vi "Main.vi"(11 "Module Admin":refnum<class "Delacor_lib_QMH_Module Admin.lvclass">) -> ()   [LabVIEW 2020, in "Data Type Scripting.lvlib"]
doc: "This template is based off of the Queued Message Handler design pattern and the Queued Message Handler project template that ships with LabVIEW.\n\nThe main difference is that the queue is private to this module and communication between modules is performed via Broadcast and Request events.\n\nRequest events are wrapped in public API methods and are handled in the Event Handling Loop (EHL) of this VI. Any module can register for Broadcast events sent by this module. The EHL generates messages based on user interface actions.\n\nThe Message Handling Loop (MHL) processes messages generated by the EHL, or by other messages. The messages are string values, so new messages can be added easily to the Message Cases case structure in the MHL. Each message cluster can also provide an optional value for Message Data, which is a variant that can be converted to whatever message-specific data is required.\n_____\nBased on DQMH Project Template 6.0.0.91."
uses:
  Data Type Scripting.lvlib
  <vilib>/Delacor/Delacor QMH/Libraries/Module Admin_class/Delacor_lib_QMH_Module Admin.lvclass
  Module Data--cluster.ctl
  _td_cluster_Settings.ctl
  Support/Poly Management/_td_map_PolyRef.ctl
  Support/Poly Management/_td_map_PolyInstanceInfo.ctl
  Support/Poly Management/_td_cluster_InstanceInfo.ctl
  <vilib>/Delacor/Delacor QMH/Libraries/Message Queue_class/Delacor_lib_QMH_Message Queue.lvclass/Delacor_lib_QMH_Message Queue.ctl
  Stop Argument--cluster.ctl
  <vilib>/Delacor/Delacor QMH/Libraries/Module Admin_class/Delacor_lib_QMH_Module Admin.lvclass/Delacor_lib_QMH_Module Admin.ctl
  Load Poly VI Argument--cluster.ctl
  Get Poly List Argument--cluster.ctl
  Get Poly Details Argument--cluster.ctl
  Open Poly VI Window Argument--cluster.ctl
  Get List of Data Types Argument--cluster.ctl
  Verify New Data Type Argument--cluster.ctl
  Create New Data Type Argument--cluster.ctl
  Edit Data Type Argument--cluster.ctl
  <vilib>/Utility/miscctls.llb/LVRectTypeDef.ctl
  Remove Data Type Argument--cluster.ctl
  Open Process Data TypeDef Argument--cluster.ctl
  Close Process Data Type Def Argument--cluster.ctl
  Edit Update Data Type Argument--cluster.ctl
  <vilib>/Delacor/Delacor QMH/Libraries/Message Queue_class/Delacor_lib_QMH_Enqueue Message (Single).vi
  <vilib>/Delacor/Delacor QMH/Libraries/Module Admin_class/Delacor_lib_QMH_Get External Launch.vi
  <vilib>/Utility/error.llb/Error Cluster From Error Code.vi
  <vilib>/ErrorRing/Error Ring.xnode
  <vilib>/Delacor/Delacor QMH/Libraries/Message Queue_class/Delacor_lib_QMH_Message Queue.lvclass
panel:
  out "error out":errorcluster
  out "Status":string
  in  "Simulate MHL Error":bool
  in  "Simulate EHL Error":bool
  # "Other QMH Modules communicate with this Module via its Public API (wrappers for its Request Events).\n\nThis Module communicates with other Modules via its Broadcast Events.\nAny module that wants to get these messages, just registers for this module's Broadcast events."
  # "This template is for the Delacor Modified Queued Message Handler design pattern.\n\nSee the block diagram for more information on how to use this template."
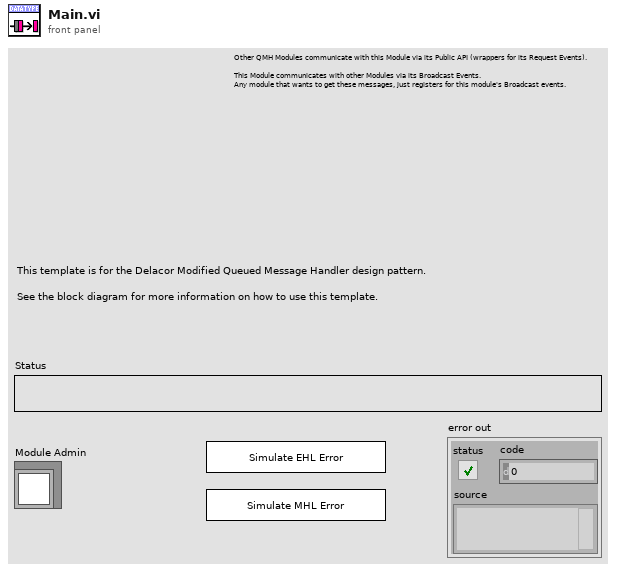
[diagram p1: front panel]
types:
  T1 = typedef "Data Type Scripting.lvlib/Request Events--cluster.ctl" = cluster{"Stop Module":refnum<user-event>, "Show Panel":refnum<user-event>, "Hide Panel":refnum<user-event>, "Get Module Execution Status":refnum<user-event>, "Show Diagram":refnum<user-event>, "Load Poly VI":refnum<user-event>, "Get Poly List":refnum<user-event>, "Get Poly Details":refnum<user-event>, "Open Poly VI Window":refnum<user-event>, "Create New Data Type":refnum<user-event>, "Verify New Data Type":refnum<user-event>, "Get List of Data Types":refnum<user-event>, "Remove Data Type":refnum<user-event>, "Open Process Data TypeDef":refnum<user-event>, "Load Edit Data Type":refnum<user-event>, "Close Process Data Type Def":refnum<user-event>, "Edit Update Data Type":refnum<user-event>}
  T2 = typedef "Data Type Scripting.lvlib/Module Data--cluster.ctl" = cluster{"Status":string, "Settings":T3, "Poly Ref Map":T4, "Poly Set Map":T5, "Valid Type?":bool, "ProcessData Ref":refnum<vi>}
  T3 = typedef "Data Type Scripting.lvlib/_td_cluster_Settings.ctl" = cluster{"NI ADAS Generic Library Path":path, "Data Types Base Directory":path, "Poly Path - Read":path, "Poly Path - Write":path, "Poly Path - Serialize":path, "Poly Path - Deserialize":path}
  T4 = typedef "_td_map_PolyRef.ctl" = map{string, refnum<vi>}
  T5 = typedef "_td_map_PolyInstanceInfo.ctl" = map{string, set{T6}}
  T6 = typedef "_td_cluster_InstanceInfo.ctl" = cluster{"VIPath":path, "Menu Name":string, "Selector Name":string}
  T7 = enum32{"invalid lock state", "Not Locked", "Locked (No Password)", "Password-protected"}
  T8 = typedef "Data Type Scripting.lvlib/Stop Argument--cluster.ctl" = cluster{"Origin":string, "Exit via Stop Module Req?":bool, "Wait for Module to stop?":bool}
  T9 = typedef "Data Type Scripting.lvlib/Load Poly VI Argument--cluster.ctl" = cluster{"Poly VI Path":path}
  T10 = typedef "Data Type Scripting.lvlib/Get Poly List Argument--cluster.ctl" = cluster{"Boolean":bool}
  T11 = typedef "Data Type Scripting.lvlib/Get Poly Details Argument--cluster.ctl" = cluster{"Poly VI Name":string}
  T12 = typedef "Data Type Scripting.lvlib/Open Poly VI Window Argument--cluster.ctl" = cluster{"Poly VI Name":string}
  T13 = typedef "Data Type Scripting.lvlib/Get List of Data Types Argument--cluster.ctl" = cluster{"Boolean":bool}
  T14 = typedef "Data Type Scripting.lvlib/Verify New Data Type Argument--cluster.ctl" = cluster{"Type Directory":path, "Type Name":string, "Menu":string, "Selector":string}
  T15 = typedef "Data Type Scripting.lvlib/Create New Data Type Argument--cluster.ctl" = cluster{"Type Directory":path, "Type Name":string, "Menu":string, "Selector":string}
  T16 = typedef "Data Type Scripting.lvlib/Edit Data Type Argument--cluster.ctl" = cluster{"Data Type":string[], "Panel Bounds":T17}
  T17 = typedef "LVRectTypeDef.ctl" = cluster{"Left":i16, "Top":i16, "Right":i16, "Bottom":i16}
  T18 = typedef "Data Type Scripting.lvlib/Remove Data Type Argument--cluster.ctl" = cluster{"Data Type to Remove":string[], "Delete Files?":bool}
  T19 = typedef "Data Type Scripting.lvlib/Open Process Data TypeDef Argument--cluster.ctl" = cluster{"Panel Bounds":T17}
  T20 = typedef "Data Type Scripting.lvlib/Close Process Data Type Def Argument--cluster.ctl" = cluster{"Boolean":bool}
  T21 = typedef "Data Type Scripting.lvlib/Edit Update Data Type Argument--cluster.ctl" = cluster{"New Data Type Name":string, "New Menu Name":string, "New Selector Name":string, "Selected Data Type":string[]}
  T22 = enum32{"Invalid", "Standard", "Closed", "Hidden", "Minimized", "Maximized"}
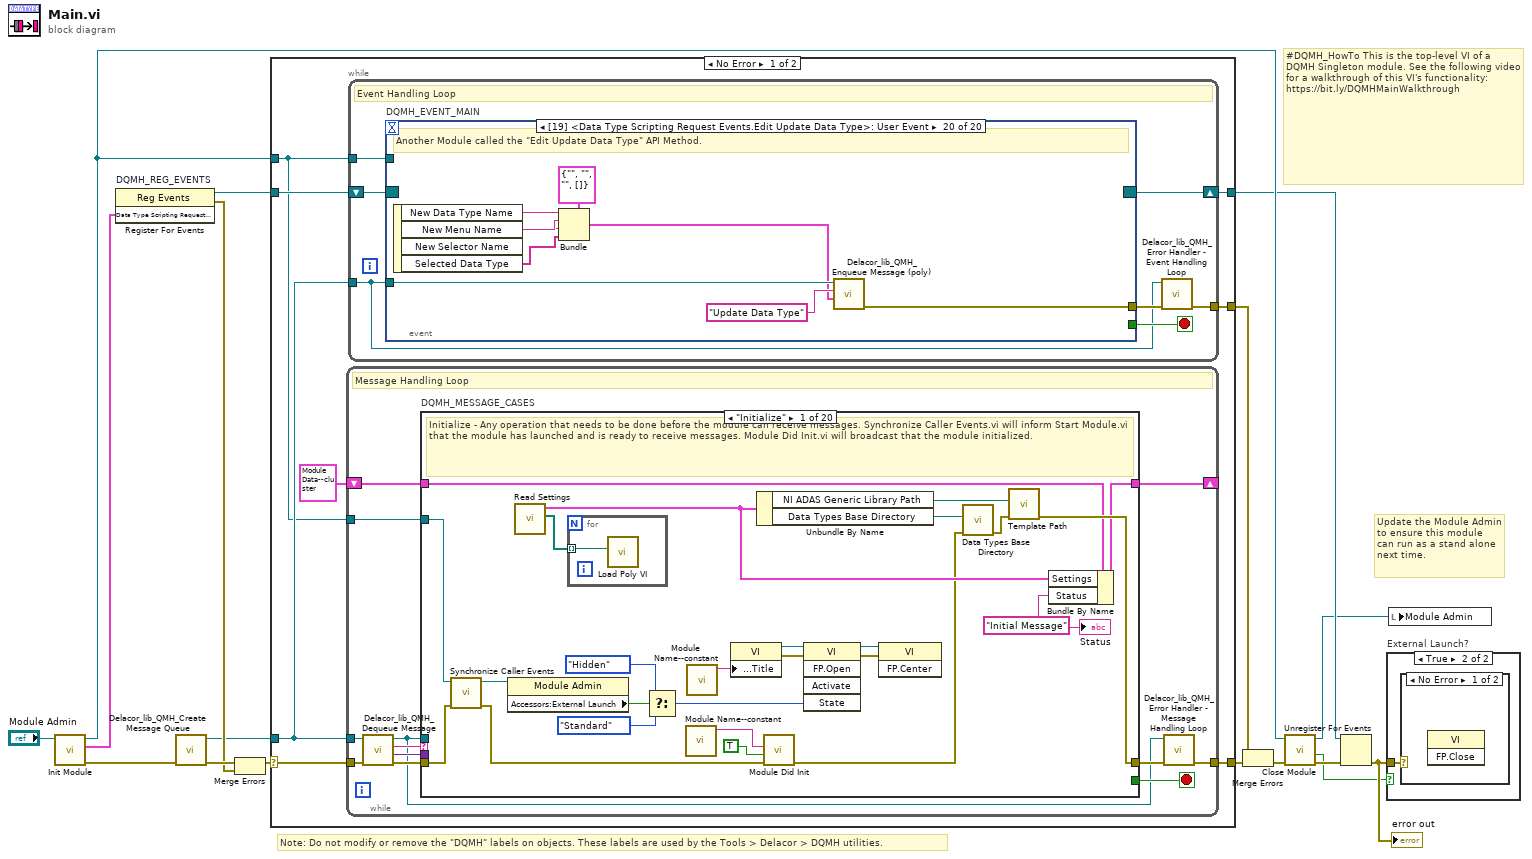
[diagram p0: block diagram]
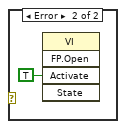
[diagram p3: hidden frame]
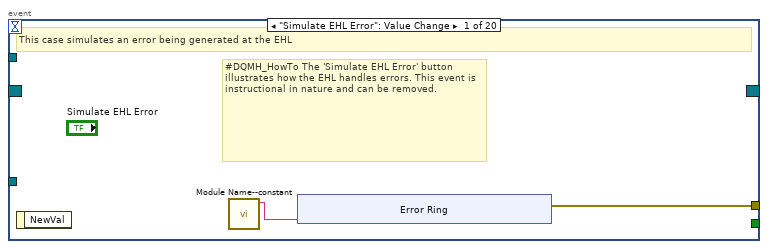
[diagram p4: hidden frame]
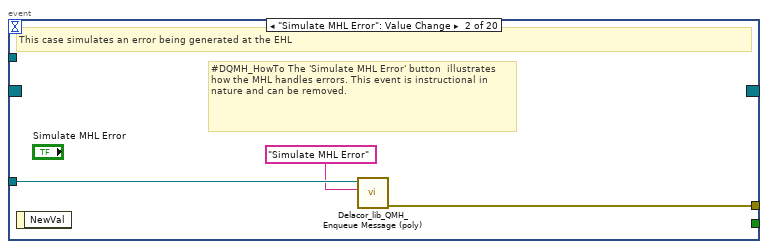
[diagram p5: hidden frame]
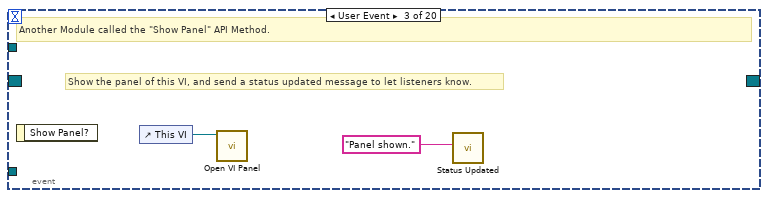
[diagram p6: hidden frame]
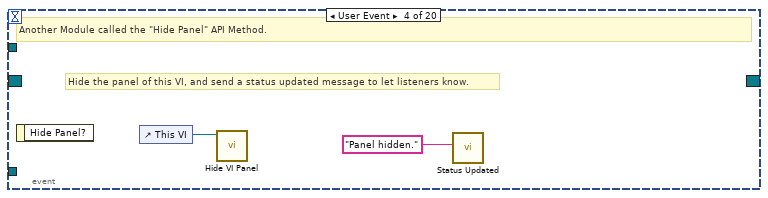
[diagram p7: hidden frame]
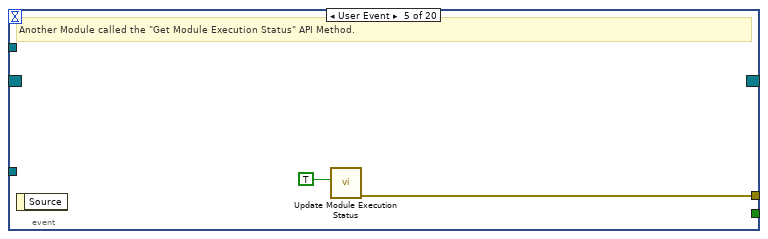
[diagram p8: hidden frame]
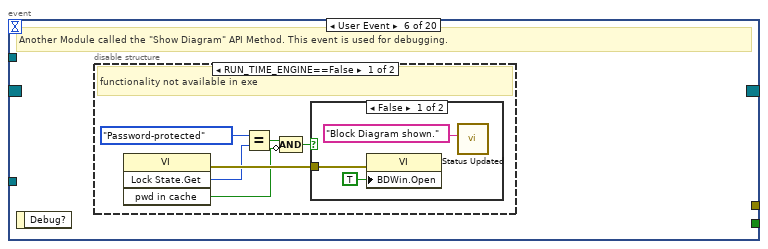
[diagram p9: hidden frame]
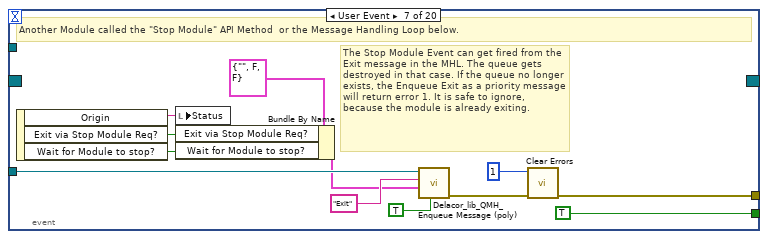
[diagram p12: hidden frame]
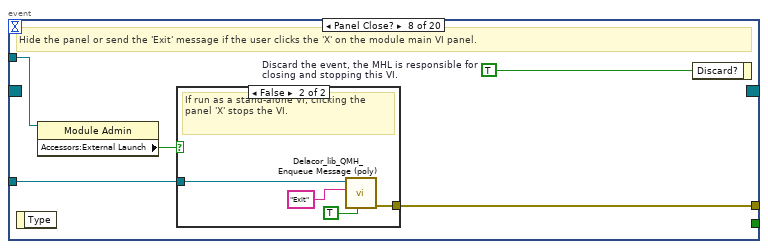
[diagram p13: hidden frame]
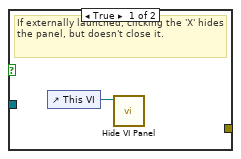
[diagram p14: hidden frame]
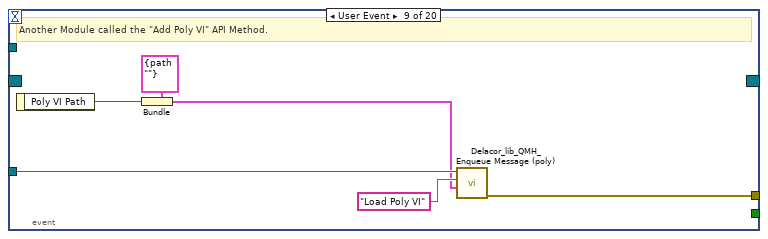
[diagram p15: hidden frame]
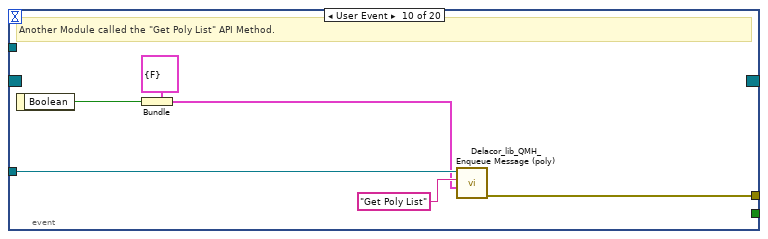
[diagram p16: hidden frame]
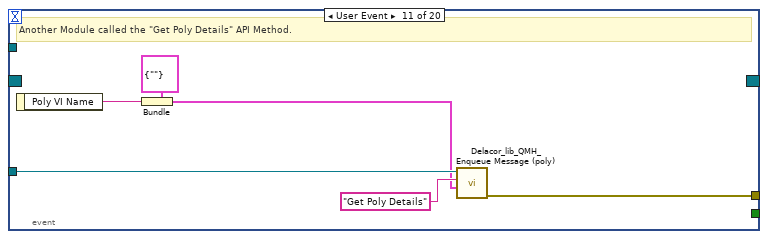
[diagram p17: hidden frame]
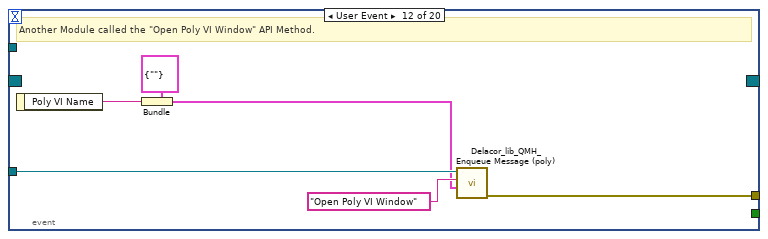
[diagram p18: hidden frame]
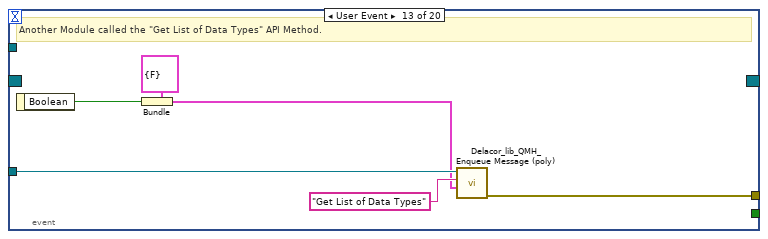
[diagram p19: hidden frame]
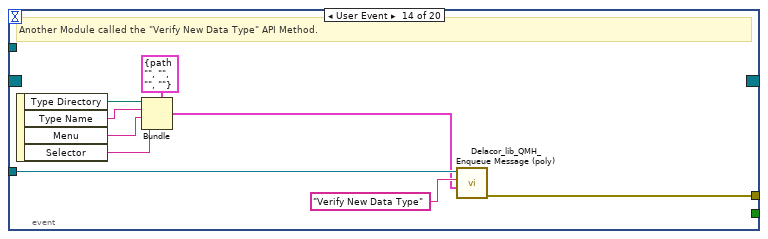
[diagram p20: hidden frame]
diagram:
  # "#DQMH_HowTo This is the top-level VI of a DQMH Singleton module. See the following video for a walkthrough of this VI's functionality: https://bit.ly/DQMHMainWalkthrough"
  # "Note: Do not modify or remove the \"DQMH\" labels on objects. These labels are used by the Tools > Delacor > DQMH utilities."
  # "Update the Module Admin to ensure this module can run as a stand alone next time."
  n1 = call "Init Module.vi"("Singleton Module Admin in"="Module Admin") -> ("error out"=w16:errorcluster, "Data Type Scripting Request Events"=w5:T1, "Singleton Module Admin out"=w8:refnum<class "Delacor_lib_QMH_Module Admin.lvclass">)  [unwired: 8 in]
  n2 = register-events "DQMH_REG_EVENTS"(w5) -> (reference out=w6:refnum<event-registration>, error out=w9:errorcluster)  [unwired: 2 in]
  n3 = call <vilib>:"Delacor_lib_QMH_Create Message Queue.vi"("error in"=w16) -> ("error out"=w11:errorcluster, "Message Queue"=w4:refnum<class "Delacor_lib_QMH_Message Queue.lvclass">)  [unwired: 9 in]
  n4 = Merge Errors(w11, w9) -> (w10:errorcluster)
  n5 = case shown="No Error" w10 {
    selector: w10 -> [w23 w477]
    tunnel: [w25 w476] -> w17
    tunnel: [w22 w482] -> w7
    tunnel: w6 -> [w20 w482]
    tunnel: w4 -> [w19 w475]
    tunnel: [w24 _] -> w14
    tunnel: w8 -> [w18 w478]
    frame No Error {
      n6 = while {
        tunnel: w19 -> [w167]
        shift-right: [w171] -> _
        shift-left: T2 {"Status"="", "Settings"={"NI ADAS Generic Library Path"=path "", "Data Types Base Directory"=path "", "Poly Path - Read"=path "", "Poly Path - Write"=path "", "Poly Path - Serialize"=path "", "Poly Path - Deserialize"=path ""}, "Poly Ref Map"={}, "Poly Set Map"={}, "Valid Type?"=FALSE, "ProcessData Ref"=refnum} ("Data Cluster") -> [w172]
        tunnel: w23 -> [w175]
        tunnel: [w173] -> w25
        tunnel: w18 -> [w165]
        stop <- w170 stop-if-true
        # "Message Handling Loop"
        n7 = call-dynamic "Delacor_lib_QMH_Dequeue Message.vi"("error in"=w175, "Message Queue in"=w167) -> ("error out"=w174:errorcluster, "Message Data"=w168:variant, "Message"=w169:string, "Message Queue out"=w166:refnum<class "Delacor_lib_QMH_Message Queue.lvclass">)  [unwired: 6 in]
        n8 = case "DQMH_MESSAGE_CASES" shown="\"Initialize\"" w169 {
          selector: w169 -> [_ _ _ _ _ _ _ _ _ _ _ _ _ _ _ _ _ _ _ w462]
          tunnel: w166 -> [_ _ _ _ _ _ _ _ _ _ _ _ _ _ _ _ _ w427 w453 _]
          tunnel: w174 -> [w198 w204 w219 w230 w246 w258 w260 w280 w292 w339 w366 w387 w392 w403 w410 w412 w417 w434 w457 w464]
          tunnel: [w201 w204 w205 w229 w237 w247 w259 w267 w291 w338 w340 w374 w394 w402 w409 w412 w416 w430 w455 w465] -> w176
          tunnel: w172 -> [w188 w203 w213 w233 w241 w254 w263 w266 w287 w321 w360 w382 w397 w401 w408 w411 w414 w429 w443 w463]
          tunnel: [w187 w203 w212 w233 w241 w254 w263 w265 w285 w326 w356 w381 w396 w400 w408 w411 w414 w429 w443 w463] -> w171
          tunnel: [_ _ _ _ _ _ _ _ _ _ _ _ _ _ _ _ _ _ w452 _] -> w170
          tunnel: w168 -> [_ _ w218 _ w245 w257 _ w279 w290 w337 w365 w386 w393 _ _ _ _ w428 w451 _]
          tunnel: w165 -> [w189 _ _ _ _ _ _ _ _ _ _ _ _ _ _ _ _ w426 w446 _]
          frame "Initialize" {
            w183 = "Initial Message" ("Initial Message")
            # "Initialize - Any operation that needs to be done before the module can receive messages. Synchronize Caller Events.vi will inform Start Module.vi that the module has launched and is ready to receive messages. Module Did Init.vi will broadcast that the module initialized."
            n9 = call "Synchronize Caller Events.vi"("error in (no error)"=w198, "Singleton Module Admin in"=w189) -> ("error out"=w197:errorcluster, "Singleton Module Admin out"=w184:refnum<class "Delacor_lib_QMH_Module Admin.lvclass">)  [unwired: 8 in]
            n10 = property class="Module Admin"(reference=w184) -> ("Accessors:External Launch"=w193:bool)  [unwired: 1 in, 2 out]
            n11 = call "Read Settings.vi"() -> ("Poly VI Paths"=w180:path[], "Settings"=w182:T3)  [unwired: 10 in]
            n12 = for {
              tunnel: w180 -> [w202] mode=indexing
              n13 = call "Load Poly VI.vi"("Poly VI Path"=w202) -> ()  [unwired: 10 in, 1 out]
            }
            n14 = Select(t=T22."Hidden" ("State"), s=w193, f=T22."Standard" ("State")) -> (s? t:f=w190:T22)
            n15 = call "Module Name--constant.vi"() -> ("Module Name"=w185:string)  [unwired: 11 in]
            n16 = call "Module Name--constant.vi"() -> ("Module Name"=w196:string)  [unwired: 11 in]
            n17 = property class="VI"("Front Panel.Title"=w196) -> (reference out=w195:refnum<vi>, error out=w200:errorcluster)  [unwired: 2 in]
            n18 = Unbundle By Name(w182) -> ("NI ADAS Generic Library Path"=w181:path, "Data Types Base Directory"=w179:path)
            n19 = call "Module Did Init.vi"("error in (no error)"=w197, "Initialized?"=TRUE, "Origin"=w185) -> ("error out"=w178:errorcluster)  [unwired: 8 in]
            n20 = invoke class="VI" method="FP.Open"(reference=w195, error in=w200, "State"=w190) -> (reference out=w194:refnum<vi>, error out=w199:errorcluster)  [unwired: 2 in, 3 out]
            n21 = invoke class="VI" method="FP.Center"(reference=w194, error in=w199) -> ()  [unwired: 1 in, 3 out]
            n22 = call "Data Types Base Directory.vi"("error in"=w178, "Data Types Directory"=w179) -> ("error out"=w177:errorcluster)  [unwired: 9 in]
            n23 = call "Template Path.vi"("error in"=w177, "Template Path"=w181) -> ("error out"=w201:errorcluster)  [unwired: 9 in]
            n24 = Bundle By Name(cluster=w188, "Settings"=w182, "Status"=w183) -> (w187:T2)
            "Status" <- w183
          }
          frame "---Module Specific---" {
            # "Separator -- The following cases handle messages specific to this Module."
          }
          frame "Load Poly VI" {
            n25 = Variant To Data(error in=w219, type=T9 {"Poly VI Path"=path ""} ("Add Poly VI Argument"), Variant=w218) -> (data=w216:T9, error out=w214:errorcluster)
            n26 = Unbundle By Name(w216) -> ("Poly VI Path"=w215:path)
            n27 = call "Open Poly VI Ref.vi"("error in"=w214, "Poly VI Path"=w215) -> ("error out"=w211:errorcluster, "Status"=w210:string, "Name"=w209:string, "Refnum out"=w208:refnum<vi>, "Success?"=w207:bool)  [unwired: 5 in]
            n28 = case shown="True" w207 {
              tunnel: w213 -> [w220 w227]
              tunnel: [w220 w226] -> w212
              tunnel: w209 -> [_ w224]
              tunnel: w208 -> [_ w221]
              frame False {
              }
              frame True {
                n29 = Unbundle By Name(w227) -> ("Poly Set Map"=w223:T5, "Poly Ref Map"=w228:T4)
                n30 = call "Poly Set Map Build.vi"("Poly Ref"=w221, "Poly Set Map in"=w223) -> ("Poly Set Map out"=w222:T5)  [unwired: 9 in]
                n31 = Insert Into Map(map in=w228, key=w224, value=w221) -> (map out=w225:T4)  [unwired: 2 out]
                n32 = Bundle By Name(cluster=w227, "Poly Set Map"=w222, "Poly Ref Map"=w225) -> (w226:T2)
              }
            }
            n33 = call "Status Updated.vi"("error in (no error)"=w211, "Status"=w210) -> ("error out"=w206:errorcluster)  [unwired: 9 in]
            n34 = call "Get Poly List.vi"("error in"=w206) -> ("error out"=w205:errorcluster)  [unwired: 10 in]
          }
          frame "Get Poly List" {
            n35 = Unbundle By Name(w233) -> ("Poly Ref Map"=w232:T4)
            n36 = for {
              tunnel: w232 -> [w236] mode=indexing
              tunnel: [w234] -> w231 mode=indexing
              n37 = Unbundle By Name(w236) -> ("Poly Ref"=w235:refnum<vi>)
              n38 = property class="PolyVI"(reference=w235) -> ("Name"=w234:string)  [unwired: 1 in, 2 out]
            }
            n39 = call "Poly List.vi"("error in"=w230, "Poly List"=w231) -> ("error out"=w229:errorcluster)  [unwired: 9 in]
          }
          frame "Get Poly Details" {
            n40 = Variant To Data(error in=w246, type=T11 {"Poly VI Name"=""} ("Get Poly Details Argument"), Variant=w245) -> (data=w243:T11, error out=w238:errorcluster)
            n41 = Unbundle By Name(w243) -> ("Poly VI Name"=w242:string)
            n42 = Unbundle By Name(w241) -> ("Poly Set Map"=w240:T5)
            n43 = call "Poly Set Map Details.vi"("Poly VI Name"=w242, "Poly Set Map in"=w240) -> ("Poly Details"=w239:T6[])  [unwired: 9 in]
            n44 = call "Poly Details.vi"("error in"=w238, "Poly Details"=w239) -> ("error out"=w237:errorcluster)  [unwired: 9 in]
          }
          frame "Open Poly VI Window" {
            n45 = Variant To Data(error in=w258, type=T12 {"Poly VI Name"=""} ("Open Poly VI Window Argument"), Variant=w257) -> (data=w255:T12, error out=w248:errorcluster)
            n46 = Unbundle By Name(w255) -> ("Poly VI Name"=w251:string)
            n47 = Unbundle By Name(w254) -> ("Poly Ref Map"=w253:T4)
            n48 = Look In Map(map=w253, key=w251) -> (value=w252:refnum<vi>)  [unwired: 1 in, 1 out]
            n49 = invoke class="PolyVI" method="FP.Open"(reference=w252) -> ()  [unwired: 4 in, 5 out]
            n50 = Format Into String(format string="Poly VI %s opened.", w251) -> (resulting string=w249:string)  [unwired: 2 in, 1 out]
            n51 = call "Status Updated.vi"("error in (no error)"=w248, "Status"=w249) -> ("error out"=w247:errorcluster)  [unwired: 9 in]
          }
          frame "Get List of Data Types" {
            n52 = Unbundle By Name(w263) -> ("Poly Set Map"=w262:T5)
            n53 = call "Poly Set Map List Data Types.vi"("Poly Set Map"=w262) -> ("Data Types"=w261:string[][])  [unwired: 10 in]
            n54 = call "List of Data Types.vi"("error in"=w260, "Data Types"=w261) -> ("error out"=w259:errorcluster)  [unwired: 9 in]
          }
          frame "Verify New Data Type" {
            n55 = Variant To Data(error in=w280, type=T14 {"Type Directory"=path "", "Type Name"="", "Menu"="", "Selector"=""} ("Verify New Data Type Argument"), Variant=w279) -> (data=w277:T14, error out=w268:errorcluster)
            n56 = Unbundle By Name(w277) -> ("Type Directory"=w276:path, "Type Name"=w275:string, "Menu"=w273:string, "Selector"=w272:string)
            n57 = Unbundle By Name(w266) -> ("Poly Set Map"=w271:T5, "Poly Ref Map"=w270:T4)
            n58 = Build Path(base path=w276, name or relative path=w275) -> (appended path=w274:path)
            n59 = call "Poly Set Map Verify New Type.vi"("Poly Set Map"=w271, "Poly Ref Map"=w270, "Selector Name"=w272, "Menu Name"=w273, "Directory"=w274) -> ("Valid?"=w264:bool, "Error Message"=w269:string)  [unwired: 5 in]
            n60 = call "Data Type Valid.vi"("error in"=w268, "Valid"=w264, "Error Msg"=w269) -> ("error out"=w267:errorcluster)  [unwired: 8 in]
            n61 = Bundle By Name(cluster=w266, "Valid Type?"=w264) -> (w265:T2)
          }
          frame "Create New Data Type" {
            n62 = Unbundle By Name(w287) -> ("Poly Ref Map"=w288:T4, "Poly Set Map"=w289:T5, "Settings.NI ADAS Generic Library Path"=w283:path, "Valid Type?"=w284:bool, "ProcessData Ref"=w282:refnum<vi>)
            n63 = case shown="True" w284 {
              tunnel: w292 -> [w295 w315]
              tunnel: [w295 w297] -> w291
              tunnel: w290 -> [_ w314]
              tunnel: w289 -> [w294 w311]
              tunnel: w288 -> [_ w310]
              tunnel: [w294 w307] -> w286
              tunnel: w283 -> [_ w306]
              tunnel: w282 -> [w293 w302]
              tunnel: [w293 refnum<vi> refnum ("ProcessData Ref")] -> w281
              frame False {
              }
              frame True {
                n64 = Variant To Data(error in=w315, type=T15 {"Type Directory"=path "", "Type Name"="", "Menu"="", "Selector"=""} ("Create New Data Type Argument"), Variant=w314) -> (data=w312:T15)  [unwired: 1 out]
                n65 = Unbundle By Name(w312) -> ("Type Directory"=w299:path, "Type Name"=w305:string, "Menu"=w308:string, "Selector"=w309:string)
                n66 = call "Copy Library.vi"("New Name"=w305, "Destination Directory"=w299, "Path to Library"=w306) -> ("error out"=w304:errorcluster, "New Library Path"=w296:path)  [unwired: 7 in]
                n67 = call "Poly Set Map Add New Type.vi"("Selector Name"=w309, "Poly Ref Map"=w310, "error in (no error)"=w304, "Menu Name"=w308, "New Library Path"=w296, "Poly Map Set in"=w311) -> ("error out"=w303:errorcluster, "Poly Map Set out"=w307:T5)  [unwired: 4 in]
                n68 = call "Save Process Data TypeDef.vi"("error in (no error)"=w303, "Path to Library"=w296, "ProcessData Ref"=w302) -> ("error out"=w300:errorcluster)  [unwired: 8 in]
                n69 = call "Update test_serialize_deserialize.vi"("error in (no error)"=w300, "Path to Library"=w296) -> ("error out"=w298:errorcluster)  [unwired: 9 in]
                n70 = call "Data Type Created.vi"("error in"=w298, "Path"=w296) -> ("error out"=w297:errorcluster)  [unwired: 9 in]
              }
            }
            n71 = Bundle By Name(cluster=w287, "Poly Set Map"=w286, "ProcessData Ref"=w281) -> (w285:T2)
          }
          frame "Load Edit Data Type" {
            n72 = Unbundle By Name(w321) -> ("ProcessData Ref"=w318:refnum<vi>)
            n73 = Variant To Data(error in=w339, type=T16 {"Data Type"=[], "Panel Bounds"={"Left"=0, "Top"=0, "Right"=0, "Bottom"=0}} ("Edit Data Type Argument"), Variant=w337) -> (data=w335:T16, error out=w338:errorcluster)
            n74 = Unbundle By Name(w335) -> ("Panel Bounds"=w316:T17, "Data Type"=w330:string[])
            n75 = invoke class="VI" method="FP.Close"(reference=w318) -> (reference out=w317:refnum<vi>)  [unwired: 2 in, 2 out]
            n76 = Close Reference(reference=w317) -> (error out=w320:errorcluster)  [unwired: 1 in]
            n77 = call <vilib>:"Clear Errors.vi"("error in (no error)"=w320) -> ("error out"=w319:errorcluster)  [unwired: 5 in, 1 out]
            n78 = Index Array(array=w330, index #1=0 ("index"), index #2=1 ("index"), index #3=2 ("index")) -> (element #1=w325:string, element #2=w324:string, element #3=w332:string)
            n79 = String To Path(string=w332) -> (path=w323:path)
            n80 = Build Path(base path=w323, name or relative path="Process Data.ctl") -> (appended path=w327:path)
            n81 = Strip Path(path=w323) -> (name=w322:string)  [unwired: 1 out]
            n82 = call "Open Process Data TypeDef.vi"("error in (no error)"=w319, "Panel Bounds"=w316, "Path to Library"=w327) -> ("ProcessData Ref"=w328:refnum<vi>)  [unwired: 7 in, 1 out]
            n83 = call "Selected Edit Data Type Info.vi"("Selector Name"=w325, "Menu Name"=w324, "Data Type Name"=w322) -> ()  [unwired: 8 in, 1 out]
            n84 = Bundle By Name(cluster=w321, "ProcessData Ref"=w328) -> (w326:T2)
          }
          frame "Update Data Type" {
            # "Don't delete if user\ndidn't change name"
            n85 = Variant To Data(error in=w366, type=T21 {"New Data Type Name"="", "New Menu Name"="", "New Selector Name"="", "Selected Data Type"=[]} ("Edit Update Data Type Argument"), Variant=w365) -> (data=w363:T21, error out=w352:errorcluster)
            n86 = Unbundle By Name(w363) -> ("Selected Data Type"=w362:string[], "New Data Type Name"=w346:string, "New Menu Name"=w355:string, "New Selector Name"=w354:string)
            n87 = Unbundle By Name(w360) -> ("Poly Ref Map"=w358:T4, "ProcessData Ref"=w353:refnum<vi>, "Poly Set Map"=w343:T5)
            n88 = call "Poly Set Map Remove Type.vi"("Poly Ref Map"=w358, "error in (no error)"=w352, "Delete Files?"=FALSE, "Data Type to Remove"=w362, "Poly Set Map in"=w343) -> ("error out"=w351:errorcluster, "Data Type Library Path"=w349:path, "Data Type Directory"=w347:path, "Poly Set Map out"=w359:T5)  [unwired: 3 in]
            n89 = call "Save Process Data TypeDef.vi"("error in (no error)"=w351, "Path to Library"=w349, "ProcessData Ref"=w353) -> ("error out"=w350:errorcluster)  [unwired: 8 in]
            n90 = Strip Path(path=w347) -> (name=w345:string)  [unwired: 1 out]
            n91 = Not Equal?(x=w346, y=w345) -> (x != y?=w344:bool)
            n92 = call "Edit - Data Type Library.vi"("Data Type Directory"=w347, "Data Type Library Path"=w349, "New Data Type Name"=w346, "error in"=w350) -> ("New Data Type Library Path"=w342:path, "Old Directory to Delete"=w348:path, "error out"=w367:errorcluster)  [unwired: 9 in]
            n93 = call "Poly Set Map Add New Type.vi"("Selector Name"=w354, "Poly Ref Map"=w358, "error in (no error)"=w367, "Menu Name"=w355, "New Library Path"=w342, "Poly Map Set in"=w359) -> ("error out"=w368:errorcluster, "Poly Map Set out"=w357:T5)  [unwired: 4 in]
            n94 = case shown="True" w344 {
              tunnel: w348 -> [_ w373]
              tunnel: w368 -> [w369 w372]
              tunnel: [w369 w371] -> w341
              frame False {
              }
              frame True {
                n95 = Delete(path (use dialog)=w373, entire hierarchy (F)=TRUE, error in=w372) -> (error out=w371:errorcluster)  [unwired: 2 in, 2 out]
              }
            }
            n96 = Bundle By Name(cluster=w360, "Poly Set Map"=w357) -> (w356:T2)
            n97 = call "Data Type Updated.vi"("error in"=w341, "Data Type Library Path"=w342) -> ("error out"=w340:errorcluster)  [unwired: 9 in]
          }
          frame "Remove Data Type" {
            n98 = Variant To Data(error in=w387, type=T18 {"Data Type to Remove"=[], "Delete Files?"=FALSE} ("Remove Data Type Argument"), Variant=w386) -> (data=w384:T18, error out=w375:errorcluster)
            n99 = Unbundle By Name(w382) -> ("Poly Ref Map"=w383:T4, "Poly Set Map"=w380:T5)
            n100 = Unbundle By Name(w384) -> ("Data Type to Remove"=w378:string[], "Delete Files?"=w377:bool)
            n101 = call "Poly Set Map Remove Type.vi"("Poly Ref Map"=w383, "error in (no error)"=w375, "Delete Files?"=w377, "Data Type to Remove"=w378, "Poly Set Map in"=w380) -> ("error out"=w376:errorcluster, "Poly Set Map out"=w379:T5)  [unwired: 3 in, 2 out]
            n102 = Bundle By Name(cluster=w382, "Poly Set Map"=w379) -> (w381:T2)
            n103 = call "Get List of Data Types.vi"("error in"=w376) -> ("error out"=w374:errorcluster)  [unwired: 10 in]
          }
          frame "Open Process Data TypeDef" {
            n104 = Variant To Data(error in=w392, type=T19 {"Panel Bounds"={"Left"=0, "Top"=0, "Right"=0, "Bottom"=0}} ("Open Process Data TypeDef Argument"), Variant=w393) -> (data=w390:T19, error out=w388:errorcluster)
            n105 = Unbundle By Name(w397) -> ("Settings.NI ADAS Generic Library Path"=w398:path)
            n106 = Unbundle By Name(w390) -> ("Panel Bounds"=w389:T17)
            n107 = call "Open Process Data TypeDef.vi"("error in (no error)"=w388, "Panel Bounds"=w389, "Path to Library"=w398) -> ("error out"=w394:errorcluster, "ProcessData Ref"=w395:refnum<vi>)  [unwired: 7 in]
            n108 = Bundle By Name(cluster=w397, "ProcessData Ref"=w395) -> (w396:T2)
          }
          frame "Close Process Data Type Def" {
            n109 = Unbundle By Name(w401) -> ("ProcessData Ref"=w404:refnum<vi>)
            n110 = invoke class="VI" method="FP.Close"(reference=w404, error in=w403) -> (reference out=w406:refnum<vi>, error out=w405:errorcluster)  [unwired: 1 in, 1 out]
            n111 = Close Reference(reference=w406, error in (no error)=w405) -> (error out=w407:errorcluster)
            n112 = call <vilib>:"Clear Errors.vi"("error in (no error)"=w407) -> ("error out"=w402:errorcluster)  [unwired: 5 in, 1 out]
            n113 = Bundle By Name(cluster=w401, "ProcessData Ref"=refnum<vi> refnum) -> (w400:T2)
          }
          frame "---Copy This Frame---" {
            # "Duplicate this frame when creating new messages.  Change this comment in the duplicated frame to describe this message."
            n114 = Merge Errors(w410) -> (w409:errorcluster)
          }
          frame "---Exit and Error Handling---" {
            # "Separator - The following cases handle errors and exit messages."
          }
          frame "Simulate MHL Error" {
            # "#DQMH_HowTo The 'Simulate MHL Error' button  illustrates how the MHL handles errors. This event is instructional in nature and can be removed."
            # "Simulate an error occurring at the MHL"
            n115 = call "Module Name--constant.vi"() -> ("Module Name"=w413:string)  [unwired: 11 in]
            n116 = xnode "Error Ring"("parameter 0"=w413) -> ("error out"=w415:errorcluster)
            n117 = Merge Errors(w417, w415) -> (w416:errorcluster)
          }
          frame "Error" {
            # "#CodeRecommended - If you ever change the name of this \"Error\" message, you'll need to update the name in the Check Loop Error.vi as well."
            # "#CodeRecommended - If the module is running in standalone mode (External Launch = FALSE), this code will pop up an error dialog and call the 'Exit' message if an error occurs. Add more fine-grained error handling here."
            # "Error - Check the error message data and respond accordingly. This message is sent by the \"Error Handler\" VIs at the end of each loop in this application."
            n118 = property class="Module Admin"(reference=w426) -> ("Accessors:External Launch"=w425:bool)  [unwired: 1 in, 2 out]
            n119 = Variant To Data(error in=w434, type=errorcluster {"status"=FALSE, "code"=0, "source"=""} ("error constant"), Variant=w428) -> (data=w435:errorcluster, error out=w432:errorcluster)
            n120 = call "Error Reported.vi"("Error"=w435) -> ()  [unwired: 10 in, 1 out]
            n121 = case shown="False" w425 {
              tunnel: [w440 _] -> w431
              tunnel: w427 -> [w438 _]
              tunnel: w435 -> [w439 _]
              frame False {
                # "If the module is running standalone, then pop up an error dialog and call the \"Exit\" message."
                n122 = call <vilib>:"Simple Error Handler.vi"("error in (no error)"=w439) -> ()  [unwired: 4 in, 5 out]
                n123 = call-poly <vilib>:"Delacor_lib_QMH_Enqueue Message (poly).vi"("Priority Message? (F)"=TRUE, "Message"="Exit", "Message Queue in"=w438) -> ("error out"=w440:errorcluster)  [unwired: 7 in, 1 out]
              }
              frame True {
                # "If the module was launched externally, calling the Error Reported broadcast VI is the only action performed by the \"Error\" message. The module's caller can then process the error appropriately."
              }
            }
            n124 = Merge Errors(w432, w431) -> (w430:errorcluster)
            n125 = local write "error out"(w430) -> ()
          }
          frame "Exit" {
            w450 = 91  # 91: not all Exit messages will have an argument
            w452 = TRUE  # Stop the VI
            # "Release the message queue reference"
            # "Exit - Exit the application."
            n126 = control-ref of="This VI"() -> (w447:refnum<vi>)
            n127 = Variant To Data(error in=w457, type=T8 {"Origin"="", "Exit via Stop Module Req?"=FALSE, "Wait for Module to stop?"=FALSE} ("Stop Argument"), Variant=w451) -> (data=w448:T8, error out=w454:errorcluster)
            n128 = call "Handle Exit.vi"("Stop Argument"=w448, "Admin in"=w446, "VI reference"=w447) -> ("error out"=w445:errorcluster)  [unwired: 7 in, 1 out]
            n129 = call <vilib>:"Clear Errors.vi"("error in (no error)"=w454, "specific error code to clear (0: all)"=w450) -> ("error out"=w456:errorcluster)  [unwired: 4 in, 1 out]
            n130 = call-dynamic "Delacor_lib_QMH_Release Message Queue.vi"("error in"=w456, "Message Queue"=w453) -> ("error out"=w444:errorcluster)  [unwired: 9 in]
            n131 = Unbundle By Name(w443) -> ("Poly Ref Map"=w442:T4)
            n132 = for {
              tunnel: w442 -> [w460] mode=indexing
              tunnel: [w458] -> w441 mode=indexing
              n133 = Unbundle By Name(w460) -> ("Poly Ref"=w459:refnum<vi>)
              n134 = Close Reference(reference=w459) -> (error out=w458:errorcluster)  [unwired: 1 in]
            }
            n135 = Merge Errors(w441, w445, w444) -> (w455:errorcluster)
          }
          frame Default {
            # "'Default' case only runs if there is a message that isn't defined in any of the other cases.  Output a programming error."
            n136 = call "Module Name--constant.vi"() -> ("Module Name"=w461:string)  [unwired: 11 in]
            n137 = xnode "Error Ring"("parameter 0"=w462, "parameter 1"=w461) -> ("error out"=w466:errorcluster)
            n138 = Merge Errors(w464, w466) -> (w465:errorcluster)
          }
        }
        n139 = call-dynamic "Delacor_lib_QMH_Error Handler - Message Handling Loop.vi"("error in"=w176, "Message Queue in"=w166) -> ("dup error in"=w173:errorcluster)  [unwired: 8 in, 1 out]
      }
      n140 = while {
        tunnel: w19 -> [w26]
        shift-right: [w29] -> w22
        shift-left: w20 -> [w30]
        tunnel: [w31] -> w24
        tunnel: w18 -> [w27]
        stop <- w28 stop-if-true
        # "Event Handling Loop"
        n141 = event "DQMH_EVENT_MAIN" shown="[19] <Data Type Scripting Request Events.Edit Update Data Type>: User Event" {
          selector: w30 -> [_ _ _ _ _ _ _ _ _ _ _ _ _ _ _ _ _ _ _ _]
          dyn-events: [_ _ _ _ _ _ _ _ _ _ _ _ _ _ _ _ _ _ _ _] -> w29
          timeout: _ -> [_ _ _ _ _ _ _ _ _ _ _ _ _ _ _ _ _ _ _ _]
          tunnel: [_ _ _ _ _ _ TRUE ("Discard?") _ _ _ _ _ _ _ _ _ _ _ _ _] -> w28
          tunnel: w26 -> [_ w43 _ _ _ _ w67 w74 w87 w93 w99 w105 w111 w120 w129 w136 w143 w149 w155 w164]
          tunnel: [w34 w44 _ _ w50 _ w70 w76 w82 w88 w94 w100 w106 w112 w121 w131 w137 w145 w150 w156] -> w32
          tunnel: w27 -> [_ _ _ _ _ _ _ w73 _ _ _ _ _ _ _ _ _ _ _ _]
          event "Simulate EHL Error": Value Change {
            # "#DQMH_HowTo The 'Simulate EHL Error' button  illustrates how the EHL handles errors. This event is instructional in nature and can be removed."
            # "This case simulates an error being generated at the EHL"
            n142 = event-data() -> ()  [unwired: 1 in, 1 out]
            n143 = call "Module Name--constant.vi"() -> ("Module Name"=w33:string)  [unwired: 11 in]
            n144 = xnode "Error Ring"("parameter 0"=w33) -> ("error out"=w34:errorcluster)
          }
          event "Simulate MHL Error": Value Change {
            # "#DQMH_HowTo The 'Simulate MHL Error' button  illustrates how the MHL handles errors. This event is instructional in nature and can be removed."
            # "This case simulates an error being generated at the EHL"
            n145 = event-data() -> ()  [unwired: 1 in, 1 out]
            n146 = call-poly <vilib>:"Delacor_lib_QMH_Enqueue Message (poly).vi"("Message"="Simulate MHL Error", "Message Queue in"=w43) -> ("error out"=w44:errorcluster)  [unwired: 8 in, 1 out]
          }
          event User Event {
            # "Show the panel of this VI, and send a status updated message to let listeners know."
            # "Another Module called the \"Show Panel\" API Method."
            n147 = event-data() -> ()  [unwired: 1 in, 1 out]
            n148 = control-ref of="This VI"() -> (w46:refnum<vi>)
            n149 = call "Open VI Panel.vi"("VI"=w46) -> ()  [unwired: 10 in, 1 out]
            n150 = call "Status Updated.vi"("Status"="Panel shown." ("format string")) -> ()  [unwired: 10 in, 1 out]
          }
          event User Event {
            # "Hide the panel of this VI, and send a status updated message to let listeners know."
            # "Another Module called the \"Hide Panel\" API Method."
            n151 = event-data() -> ()  [unwired: 1 in, 1 out]
            n152 = control-ref of="This VI"() -> (w48:refnum<vi>)
            n153 = call "Hide VI Panel.vi"("VI"=w48) -> ()  [unwired: 10 in, 1 out]
            n154 = call "Status Updated.vi"("Status"="Panel hidden." ("format string")) -> ()  [unwired: 10 in, 1 out]
          }
          event User Event {
            # "Another Module called the \"Get Module Execution Status\" API Method."
            n155 = event-data() -> ()  [unwired: 1 in, 1 out]
            n156 = call "Update Module Execution Status.vi"("Running?"=TRUE) -> ("error out"=w50:errorcluster)  [unwired: 10 in]
          }
          event User Event {
            # "Another Module called the \"Show Diagram\" API Method. This event is used for debugging."
            n157 = event-data() -> ()  [unwired: 1 in, 1 out]
            n158 = disable-structure shown="RUN_TIME_ENGINE==False" {
              frame condition #0 (active) {
                # "functionality not available in exe"
                n159 = invoke class="VI" method="Lock State.Get"() -> (error out=w56:errorcluster, "Get Lock State"=w55:T7, "pwd in cache"=w52:bool)  [unwired: 4 in, 1 out]
                n160 = Equal?(x=T7."Password-protected", y=w55) -> (x = y?=w53:bool)
                n161 = Compound Arithmetic op=AND(w53, invert w52) -> (w51:bool)
                n162 = case shown="False" w51 {
                  tunnel: w56 -> [w59 _]
                  frame False {
                    n163 = property class="VI"(error in=w59, "BDWin.Open"=TRUE ("Block Diagram Window:Open")) -> ()  [unwired: 1 in, 2 out]
                    n164 = call "Status Updated.vi"("Status"="Block Diagram shown." ("format string")) -> ()  [unwired: 10 in, 1 out]
                  }
                  frame True {
                    # "Password-protected VI, and the password is not in the cache. Do not show the diagram."
                  }
                }
              }
              frame condition #1 {
              }
            }
          }
          event User Event {
            # "The Stop Module Event can get fired from the Exit message in the MHL. The queue gets destroyed in that case. If the queue no longer exists, the Enqueue Exit as a priority message will return error 1. It is safe to ignore, because the module is already exiting."
            # "Another Module called the \"Stop Module\" API Method  or the Message Handling Loop below."
            n165 = event-data() -> ("Origin"=w66:string, "Exit via Stop Module Req?"=w62:bool, "Wait for Module to stop?"=w61:bool)  [unwired: 1 in]
            n166 = local write "Status"(w66) -> ()
            n167 = Bundle By Name(cluster=T8 {"Origin"="", "Exit via Stop Module Req?"=FALSE, "Wait for Module to stop?"=FALSE} ("Stop Argument"), "Exit via Stop Module Req?"=w62, "Wait for Module to stop?"=w61) -> (w60:T8)
            n168 = call-poly <vilib>:"Delacor_lib_QMH_Enqueue Message (poly).vi"("Priority Message? (F)"=TRUE, "Message Data"=w60, "Message"="Exit", "Message Queue in"=w67) -> ("error out"=w71:errorcluster)  [unwired: 6 in, 1 out]
            n169 = call <vilib>:"Clear Errors.vi"("error in (no error)"=w71, "specific error code to clear (0: all)"=1) -> ("error out"=w70:errorcluster)  [unwired: 4 in, 1 out]
          }
          event Panel Close? {
            w75 = TRUE  # Discard the event, the MHL is responsible for closing and stopping this VI.
            # "Hide the panel or send the 'Exit' message if the user clicks the 'X' on the module main VI panel."
            n170 = event-data() -> ()  [unwired: 1 in, 1 out]
            n171 = property class="Module Admin"(reference=w73) -> ("Accessors:External Launch"=w72:bool)  [unwired: 1 in, 2 out]
            n172 = case shown="False" w72 {
              tunnel: w74 -> [_ w80]
              tunnel: [_ w81] -> w76
              frame True {
                # "If externally launched, clicking the 'X' hides the panel, but doesn't close it."
                n173 = control-ref of="This VI"() -> (w77:refnum<vi>)
                n174 = call "Hide VI Panel.vi"("VI"=w77) -> ()  [unwired: 10 in, 1 out]
              }
              frame False {
                # "If run as a stand-alone VI, clicking the panel 'X' stops the VI."
                n175 = call-poly <vilib>:"Delacor_lib_QMH_Enqueue Message (poly).vi"("Priority Message? (F)"=TRUE, "Message"="Exit", "Message Queue in"=w80) -> ("error out"=w81:errorcluster)  [unwired: 7 in, 1 out]
              }
            }
            n176 = event-data("Discard?"=w75) -> ()  [unwired: 1 in, 1 out]
          }
          event User Event {
            # "Another Module called the \"Add Poly VI\" API Method."
            n177 = event-data() -> ("Poly VI Path"=w83:path)  [unwired: 1 in]
            n178 = Bundle(cluster=T9 {"Poly VI Path"=path ""} ("Add Poly VI Argument"), "Poly VI Path"=w83) -> (w84:T9)
            n179 = call-poly <vilib>:"Delacor_lib_QMH_Enqueue Message (poly).vi"("Message Data"=w84, "Message"="Load Poly VI", "Message Queue in"=w87) -> ("error out"=w82:errorcluster)  [unwired: 7 in, 1 out]
          }
          event User Event {
            # "Another Module called the \"Get Poly List\" API Method."
            n180 = event-data() -> ("Boolean"=w89:bool)  [unwired: 1 in]
            n181 = Bundle(cluster=T10 {"Boolean"=FALSE} ("Get Poly List Argument"), "Boolean"=w89) -> (w90:T10)
            n182 = call-poly <vilib>:"Delacor_lib_QMH_Enqueue Message (poly).vi"("Message Data"=w90, "Message"="Get Poly List", "Message Queue in"=w93) -> ("error out"=w88:errorcluster)  [unwired: 7 in, 1 out]
          }
          event User Event {
            # "Another Module called the \"Get Poly Details\" API Method."
            n183 = event-data() -> ("Poly VI Name"=w95:string)  [unwired: 1 in]
            n184 = Bundle(cluster=T11 {"Poly VI Name"=""} ("Get Poly Details Argument"), "Poly VI Name"=w95) -> (w96:T11)
            n185 = call-poly <vilib>:"Delacor_lib_QMH_Enqueue Message (poly).vi"("Message Data"=w96, "Message"="Get Poly Details", "Message Queue in"=w99) -> ("error out"=w94:errorcluster)  [unwired: 7 in, 1 out]
          }
          event User Event {
            # "Another Module called the \"Open Poly VI Window\" API Method."
            n186 = event-data() -> ("Poly VI Name"=w101:string)  [unwired: 1 in]
            n187 = Bundle(cluster=T12 {"Poly VI Name"=""} ("Open Poly VI Window Argument"), "Poly VI Name"=w101) -> (w102:T12)
            n188 = call-poly <vilib>:"Delacor_lib_QMH_Enqueue Message (poly).vi"("Message Data"=w102, "Message"="Open Poly VI Window", "Message Queue in"=w105) -> ("error out"=w100:errorcluster)  [unwired: 7 in, 1 out]
          }
          event User Event {
            # "Another Module called the \"Get List of Data Types\" API Method."
            n189 = event-data() -> ("Boolean"=w107:bool)  [unwired: 1 in]
            n190 = Bundle(cluster=T13 {"Boolean"=FALSE} ("Get List of Data Types Argument"), "Boolean"=w107) -> (w108:T13)
            n191 = call-poly <vilib>:"Delacor_lib_QMH_Enqueue Message (poly).vi"("Message Data"=w108, "Message"="Get List of Data Types", "Message Queue in"=w111) -> ("error out"=w106:errorcluster)  [unwired: 7 in, 1 out]
          }
          event User Event {
            # "Another Module called the \"Verify New Data Type\" API Method."
            n192 = event-data() -> ("Type Directory"=w116:path, "Type Name"=w115:string, "Menu"=w114:string, "Selector"=w113:string)  [unwired: 1 in]
            n193 = Bundle(cluster=T14 {"Type Directory"=path "", "Type Name"="", "Menu"="", "Selector"=""} ("Verify New Data Type Argument"), "Type Directory"=w116, "Type Name"=w115, "Menu"=w114, "Selector"=w113) -> (w117:T14)
            n194 = call-poly <vilib>:"Delacor_lib_QMH_Enqueue Message (poly).vi"("Message Data"=w117, "Message"="Verify New Data Type", "Message Queue in"=w120) -> ("error out"=w112:errorcluster)  [unwired: 7 in, 1 out]
          }
          event User Event {
            # "Another Module called the \"Create New Data Type\" API Method."
            n195 = event-data() -> ("Type Directory"=w125:path, "Type Name"=w124:string, "Menu"=w123:string, "Selector"=w122:string)  [unwired: 1 in]
            n196 = Bundle(cluster=T15 {"Type Directory"=path "", "Type Name"="", "Menu"="", "Selector"=""} ("Create New Data Type Argument"), "Type Directory"=w125, "Type Name"=w124, "Menu"=w123, "Selector"=w122) -> (w126:T15)
            n197 = call-poly <vilib>:"Delacor_lib_QMH_Enqueue Message (poly).vi"("Message Data"=w126, "Message"="Create New Data Type", "Message Queue in"=w129) -> ("error out"=w121:errorcluster)  [unwired: 7 in, 1 out]
          }
          event User Event {
            # "Another Module called the \"Edit Data Type\" API Method."
            n198 = event-data() -> ("Data Type"=w132:string[], "Panel Bounds"=w130:T17)  [unwired: 1 in]
            n199 = Bundle(cluster=T16 {"Data Type"=[], "Panel Bounds"={"Left"=0, "Top"=0, "Right"=0, "Bottom"=0}} ("Edit Data Type Argument"), "Data Type"=w132, "Panel Bounds"=w130) -> (w133:T16)
            n200 = call-poly <vilib>:"Delacor_lib_QMH_Enqueue Message (poly).vi"("Message Data"=w133, "Message"="Load Edit Data Type", "Message Queue in"=w136) -> ("error out"=w131:errorcluster)  [unwired: 7 in, 1 out]
          }
          event User Event {
            # "Another Module called the \"Remove Data Type\" API Method."
            n201 = event-data() -> ("Data Type to Remove"=w139:string[], "Delete Files?"=w138:bool)  [unwired: 1 in]
            n202 = Bundle(cluster=T18 {"Data Type to Remove"=[], "Delete Files?"=FALSE} ("Remove Data Type Argument"), "Data Type to Remove"=w139, "Delete Files?"=w138) -> (w140:T18)
            n203 = call-poly <vilib>:"Delacor_lib_QMH_Enqueue Message (poly).vi"("Message Data"=w140, "Message"="Remove Data Type", "Message Queue in"=w143) -> ("error out"=w137:errorcluster)  [unwired: 7 in, 1 out]
          }
          event User Event {
            # "Another Module called the \"Open Process Data TypeDef\" API Method."
            n204 = event-data() -> ("Panel Bounds"=w144:T17)  [unwired: 1 in]
            n205 = Bundle(cluster=T19 {"Panel Bounds"={"Left"=0, "Top"=0, "Right"=0, "Bottom"=0}} ("Open Process Data TypeDef Argument"), "Panel Bounds"=w144) -> (w146:T19)
            n206 = call-poly <vilib>:"Delacor_lib_QMH_Enqueue Message (poly).vi"("Message Data"=w146, "Message"="Open Process Data TypeDef", "Message Queue in"=w149) -> ("error out"=w145:errorcluster)  [unwired: 7 in, 1 out]
          }
          event User Event {
            # "Another Module called the \"Close Process Data Type Def\" API Method."
            n207 = event-data() -> ("Boolean"=w151:bool)  [unwired: 1 in]
            n208 = Bundle(cluster=T20 {"Boolean"=FALSE} ("Close Process Data Type Def Argument"), "Boolean"=w151) -> (w152:T20)
            n209 = call-poly <vilib>:"Delacor_lib_QMH_Enqueue Message (poly).vi"("Message Data"=w152, "Message"="Close Process Data Type Def", "Message Queue in"=w155) -> ("error out"=w150:errorcluster)  [unwired: 7 in, 1 out]
          }
          event User Event {
            # "Another Module called the \"Edit Update Data Type\" API Method."
            n210 = event-data() -> ("New Data Type Name"=w160:string, "New Menu Name"=w159:string, "New Selector Name"=w158:string, "Selected Data Type"=w157:string[])  [unwired: 1 in]
            n211 = Bundle(cluster=T21 {"New Data Type Name"="", "New Menu Name"="", "New Selector Name"="", "Selected Data Type"=[]} ("Edit Update Data Type Argument"), "New Data Type Name"=w160, "New Menu Name"=w159, "New Selector Name"=w158, "Selected Data Type"=w157) -> (w161:T21)
            n212 = call-poly <vilib>:"Delacor_lib_QMH_Enqueue Message (poly).vi"("Message Data"=w161, "Message"="Update Data Type", "Message Queue in"=w164) -> ("error out"=w156:errorcluster)  [unwired: 7 in, 1 out]
          }
        }
        n213 = call-dynamic "Delacor_lib_QMH_Error Handler - Event Handling Loop.vi"("error in"=w32, "Message Queue in"=w26) -> ("dup error in"=w31:errorcluster)  [unwired: 8 in, 1 out]
      }
    }
    frame Error {
      # "Synchronize Caller Events.vi will inform Start Module.vi that the module has launched and will let the code calling Start Module.vi register for broadcasts and would permit the caller receive the broadcast that an error occurred at launch time."
      n214 = call-dynamic "Delacor_lib_QMH_Release Message Queue.vi"("error in"=w477, "Message Queue"=w475) -> ("error out"=w476:errorcluster)  [unwired: 9 in]
      n215 = call "Synchronize Caller Events.vi"("Singleton Module Admin in"=w478) -> ("error out"=w483:errorcluster)  [unwired: 9 in, 1 out]
      n216 = call "Module Name--constant.vi"() -> ("Module Name"=w481:string)  [unwired: 11 in]
      n217 = Format Into String(format string="An error occurred during initialization. %s is no longer running.", w481) -> (resulting string=w479:string)  [unwired: 2 in, 1 out]
      n218 = Merge Errors(w476, w483) -> (w484:errorcluster)
      n219 = call "Error Reported.vi"("Additional Information"=w479, "Error"=w484) -> ()  [unwired: 9 in, 1 out]
    }
  }
  n220 = Merge Errors(w14, w17) -> (w13:errorcluster)
  n221 = call "Close Module.vi"("error in (no error)"=w13, "Module Admin in"=w8) -> ("error out"=w15:errorcluster, "External Launch"=w1:bool, "Module Admin out"=w2:refnum<class "Delacor_lib_QMH_Module Admin.lvclass">)  [unwired: 7 in]
  n222 = Unregister For Events(event registration refnum=w7, error in=w15) -> (error out=w12:errorcluster)
  "error out" <- w12
  n223 = case "External Launch?" shown="True" w1 {
    tunnel: w12 -> [_ w485]
    frame False {
    }
    frame True {
      n224 = case shown="No Error" w485 {
        frame No Error {
          n225 = invoke class="VI" method="FP.Close"() -> ()  [unwired: 3 in, 3 out]
        }
        frame Error {
          n226 = invoke class="VI" method="FP.Open"("Activate"=TRUE ("Activate?")) -> ()  [unwired: 4 in, 5 out]
        }
      }
    }
  }
  n227 = local write "Module Admin"(w2) -> ()
